vi "sub vi - send mail v3.vi"(0 "TO:":string, 5 "message":string, 7 "subject":string, 9 "out going server":string, 11 "from":string, 12 "username":string, 13 "password":string) -> (15 "error out":errorcluster)   [LabVIEW 2013]
uses:
  <vilib>/smtpClient/Set Message Text.vi
  <vilib>/smtpClient/LabVIEWSMTPClient.lvlib
panel:
  in  "Tab Control":enum32{"Page 1", "Page 2"}(tab)
  in  "Array - send address string":string[](array[string])
  # "SENDING MAIL TO:"
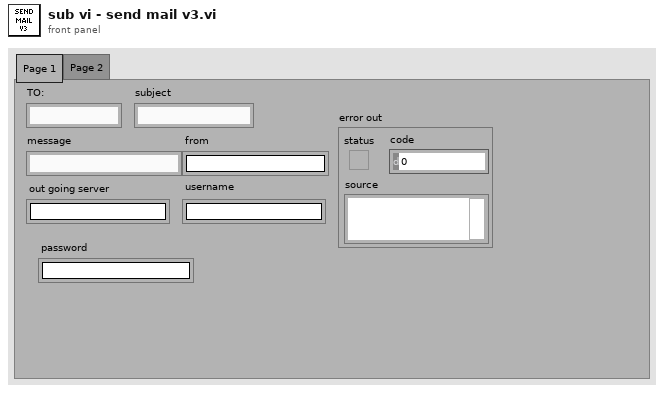
[diagram p1: front panel]
types:
  T1 = typedef "LabVIEWSMTPClient.lvlib/SmtpClientHandle.ctl" = refnum<k1>
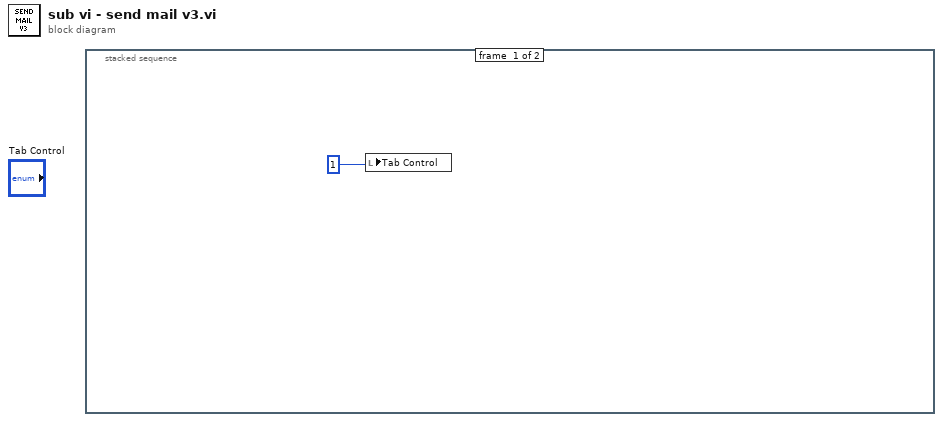
[diagram p0: block diagram]
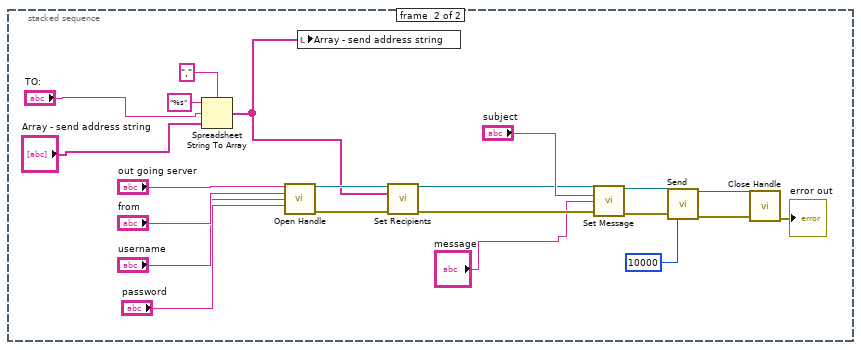
[diagram p2: hidden frame]
diagram:
  n1 = stacked-sequence {
    frame #0 {
      n2 = local write "Tab Control"(1) -> ()
    }
    frame #1 {
      n3 = Spreadsheet String To Array(delimiter (Tab)=",", format string="%s", spreadsheet string="TO:", array type (2D Dbl)="Array - send address string") -> (array=w9:string[])
      n4 = call <vilib>:"Open Handle.vi"("server address"="out going server", "from"="from", "username"="username", "password"="password") -> ("handle out"=w22:T1, "error out"=w21:errorcluster)  [unwired: 10 in]
      n5 = local write "Array - send address string"(w9) -> ()
      n6 = call <vilib>:"Set Recipients.vi"("handle in"=w22, "to"=w9, "error in (no error)"=w21) -> ("handle out"=w4:T1, "error out"=w3:errorcluster)  [unwired: 11 in]
      n7 = call-poly <vilib>:"Set Message.vi"("handle in"=w4, "subject"="subject", "plain text message"="message", "error in (no error)"=w3) -> ("handle out"=w19:T1, "error out"=w18:errorcluster)  [unwired: 10 in]
      n8 = call <vilib>:"Send.vi"("handle in"=w19, "error in (no error)"=w18, "timeout in ms (10000)"=10000) -> ("handle out"=w17:T1, "error out"=w16:errorcluster)  [unwired: 10 in, 1 out]
      n9 = call <vilib>:"Close Handle.vi"("handle in"=w17, "error in (no error)"=w16) -> ("error out"=→"error out":errorcluster)  [unwired: 12 in, 1 out]
    }
  }
